vi "Untitled 1.vi"() -> ()   [LabVIEW 2020]
uses:
  <vilib>/Instr/_visa.llb/VISA Configure Serial Port (Instr).vi
panel:
  in  "Enviar":bool
  in  "B1":bool
  in  "B0":bool
  out "A0":bool
  out "Thermometer":dbl(slide) scale=0.0..500.0
  out "A1":bool
  out "read buffer":string
  in  "stop":bool
  in  "VISA resource name":refnum<visa-resource-name>
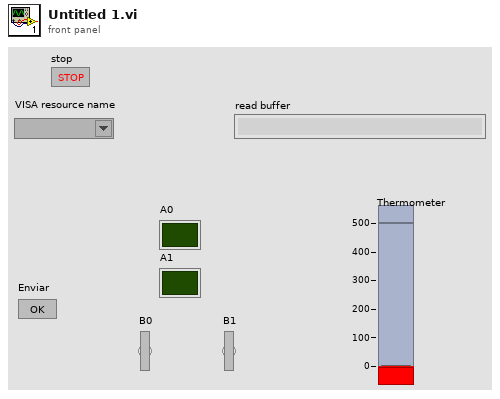
[diagram p1: front panel]
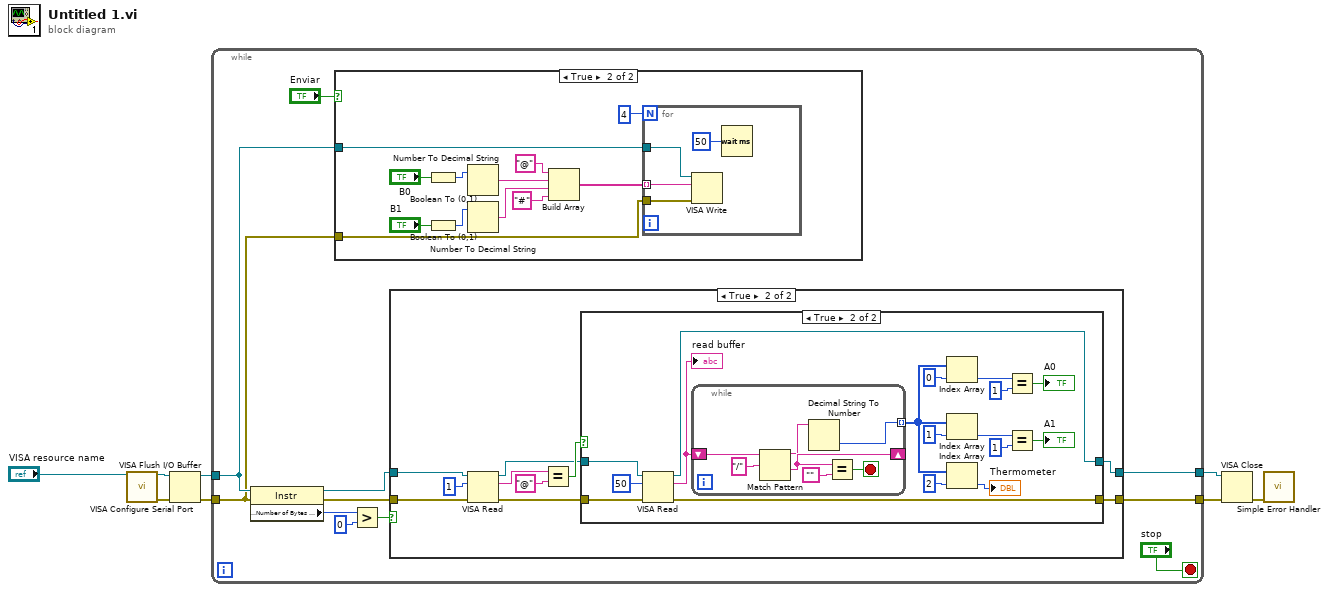
[diagram p0: block diagram]
diagram:
  n1 = call-poly "VISA Configure Serial Port"("VISA resource name"="VISA resource name") -> ("VISA resource name out"=w6:refnum<visa-resource-name>, "error out"=w7:errorcluster)  [unwired: 13 in]
  n2 = VISA Flush I/O Buffer(VISA resource name=w6, error in (no error)=w7) -> (VISA resource name out=w5:refnum<visa-resource-name>, error out=w4:errorcluster)  [unwired: 1 in]
  n3 = while {
    tunnel: w5 -> [w10]
    tunnel: w4 -> [w9]
    tunnel: [w13] -> w2
    tunnel: [w12] -> w3
    stop <- "stop" stop-if-true
    n4 = property class="Instr"(reference=w10, error in=w9) -> (reference out=w15:refnum<visa-resource-name>, error out=w14:errorcluster, "Serial Settings:Number of Bytes at Serial Port"=w18:u32)
    n5 = case shown="True" "Enviar" {
      tunnel: w10 -> [_ w21]
      tunnel: w9 -> [_ w20]
      frame False {
      }
      frame True {
        n6 = Boolean To (0,1)(Boolean="B0") -> (0, 1=w25:i16)
        n7 = Boolean To (0,1)(Boolean="B1") -> (0, 1=w28:i16)
        n8 = Number To Decimal String(number=w25) -> (decimal integer string=w24:string)  [unwired: 1 in]
        n9 = Number To Decimal String(number=w28) -> (decimal integer string=w27:string)  [unwired: 1 in]
        n10 = Build Array("@", w24, w27, "#") -> (w22:string[])
        n11 = for {
          N: 4 -> [_]
          tunnel: w22 -> [w35] mode=indexing
          tunnel: w21 -> [w34]
          tunnel: w20 -> [w33]
          n12 = VISA Write(VISA resource name=w34, write buffer=w35, error in (no error)=w33) -> ()  [unwired: 3 out]
          n13 = Wait (ms)(milliseconds to wait=u32 50) -> ()  [unwired: 1 out]
        }
      }
    }
    n14 = Greater?(x=w18, y=u32 0) -> (0:w16:bool)
    n15 = case shown="True" w16 {
      tunnel: w15 -> [w37 w47]
      tunnel: w14 -> [w36 w46]
      tunnel: [w37 w39] -> w13
      tunnel: [w36 w38] -> w12
      frame False {
      }
      frame True {
        n16 = VISA Read(VISA resource name=w47, byte count=u32 1, error in (no error)=w46) -> (VISA resource name out=w41:refnum<visa-resource-name>, read buffer=w44:string, error out=w40:errorcluster)  [unwired: 1 out]
        n17 = Equal?(x=w44, y="@") -> (x = y?=w42:bool)
        n18 = case shown="True" w42 {
          tunnel: w41 -> [w49 w66]
          tunnel: w40 -> [w48 w65]
          tunnel: [w49 w63] -> w39
          tunnel: [w48 w62] -> w38
          frame False {
          }
          frame True {
            n19 = VISA Read(VISA resource name=w66, byte count=u32 50, error in (no error)=w65) -> (VISA resource name out=w63:refnum<visa-resource-name>, read buffer=w61:string, error out=w62:errorcluster)  [unwired: 1 out]
            "read buffer" <- w61
            n20 = while {
              shift-right: [w71] -> _
              shift-left: w61 -> [w72]
              tunnel: [w67] -> w54 mode=indexing
              stop <- w69 stop-if-true
              n21 = Match Pattern(string=w72, regular expression="/") -> (before substring=w68:string, after substring=w71:string)  [unwired: 1 in, 2 out]
              n22 = Decimal String To Number(string=w68) -> (number=w67:i32)  [unwired: 2 in, 1 out]
              n23 = Equal?(x=w71, y="") -> (x = y?=w69:bool)
            }
            n24 = Index Array(array=w54, index=0) -> (element=w50:i32)
            n25 = Index Array(array=w54, index=1) -> (element=w52:i32)
            n26 = Index Array(array=w54, index=2) -> (element=→"Thermometer":i32)
            n27 = Equal?(x=w50, y=1) -> (x = y?=→"A0":bool)
            n28 = Equal?(x=w52, y=1) -> (x = y?=→"A1":bool)
          }
        }
      }
    }
  }
  n29 = VISA Close(VISA resource name=w2, error in (no error)=w3) -> (error out=w1:errorcluster)
  n30 = call <vilib>:"Simple Error Handler.vi"("error in (no error)"=w1) -> ()  [unwired: 4 in, 5 out]
